vi "Status Get User Compensation.vi"(5 "Retry Attempts (0)":i32 min=0, 7 "Fast Comms (F)":bool, 8 "error in":errorcluster, 11 "VISA resource name":refnum<visa-resource-name>) -> (0 "error out":errorcluster, 2 "User Compensation":dbl format="%#_6f", 3 "VISA resource name out":refnum<visa-resource-name>)   [LabVIEW 2020, in "driver_chromtech_next_gen.lvlib"]
doc: "Returns the user flow rate compensation."
uses:
  driver_chromtech_next_gen.lvlib
panel:
  out "Response":string
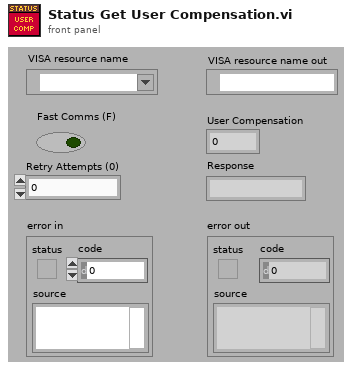
[diagram p1: front panel]
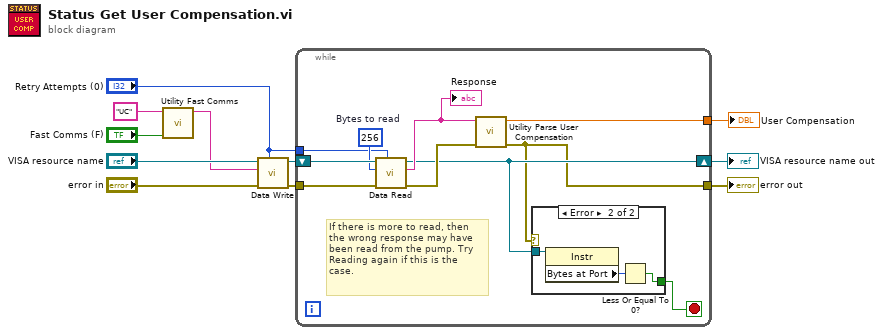
[diagram p0: block diagram]
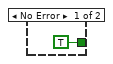
[diagram p2: hidden frame]
diagram:
  n1 = call "Utility Fast Comms.vi"("Fast Comms"="Fast Comms (F)", "Command"="UC") -> ("Fast Command"=w9:string)  [unwired: 9 in]
  n2 = call "Data Write.vi"("Retry Attempts (0)"="Retry Attempts (0)", "error in (no error)"="error in", "Command"=w9, "VISA Refnum in"="VISA resource name") -> ("error out"=w6:errorcluster, "VISA Refnum out"=w5:refnum<visa-resource-name>)  [unwired: 6 in]
  n3 = while {
    tunnel: [w20] -> w7
    tunnel: "Retry Attempts (0)" -> [w15]
    shift-right: [w14] -> w2
    shift-left: w5 -> [w18]
    tunnel: w6 -> [w19]
    tunnel: [w13] -> w1
    stop <- w12 stop-if-true
    w17 = u32 256  # Bytes to read
    # "If there is more to read, then\nthe wrong response may have\nbeen read from the pump. Try\nReading again if this is the\ncase."
    n4 = call "Data Read.vi"("Retry Attempts (0)"=w15, "error in (no error)"=w19, "Bytes to read"=w17, "VISA Refnum in"=w18) -> ("error out"=w21:errorcluster, "read buffer"=w16:string, "VISA Refnum out"=w14:refnum<visa-resource-name>)  [unwired: 5 in]
    "Response" <- w16
    n5 = call "Utility Parse User Compensation.vi"("error in (no error)"=w21, "Input String"=w16) -> ("error out"=w13:errorcluster, "Compensation"=w20:dbl)  [unwired: 8 in]
    n6 = case shown="Error" w13 {
      tunnel: w14 -> [_ w25]
      tunnel: [TRUE w23] -> w12
      frame No Error {
      }
      frame Error {
        n7 = property class="Instr"(reference=w25) -> ("Bytes at Port"=w24:u32)  [unwired: 1 in, 2 out]
        n8 = Less Or Equal To 0?(x=w24) -> (x <= 0?=w23:bool)
      }
    }
  }
  "VISA resource name out" <- w2
  "error out" <- w1
  "User Compensation" <- w7
